vi "take_i64_from_BSON_bytes.vi"(11 "BSONbytes":u8[](array[numeric])) -> (2 "restOfBytes":u8[](array[numeric]), 3 "value":i64)   [LabVIEW 2015, in "BSON_convertors_Library.lvlib"]
uses:
  BSON_convertors_Library.lvlib
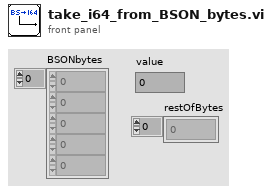
[diagram p1: front panel]
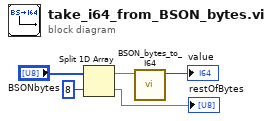
[diagram p0: block diagram]
diagram:
  n1 = Split 1D Array(array="BSONbytes", index=8) -> (first subarray=w2:u8[], second subarray=→"restOfBytes":u8[])
  n2 = call "BSON_bytes_to_I64.vi"("BSONbytes"=w2) -> ("value"=→"value":i64)  [unwired: 10 in]
